vi "ExSubBin2x.vi"(2 "error in (no error)":errorcluster, 3 "Camera Handle":u32) -> (0 "error out":errorcluster, 1 "Camera Handle":u32)   [LabVIEW 2010]
panel:
  # "This is a SubVI that bins the CCD chip\nby 2 in both the x and y dimensions."
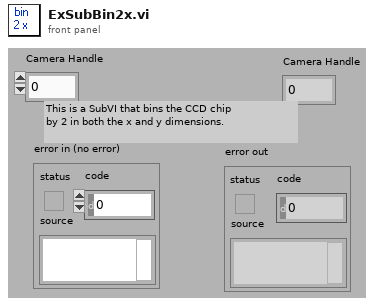
[diagram p1: front panel]
types:
  T1 = cluster{"X start":u32, "X end":u32, "X Binning/Grouping":u32, "Y start":u32, "Y end":u32, "Y Binning/Grouping":u32}
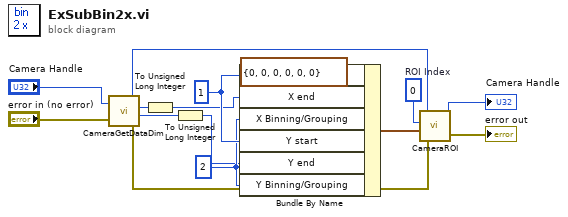
[diagram p0: block diagram]
diagram:
  w8 = u32 0  # ROI Index
  w6 = u32 2
  w7 = u32 1
  n1 = call <userlib>:"CameraGetDataDim.vi"("Camera Handle"="Camera Handle", "error in"="error in (no error)") -> ("Camera Handle"=w14:u32, "Xdim"=w5:u32, "Ydim"=w3:u32, "error out"=w12:errorcluster)
  n2 = To Unsigned Long Integer(number=w5) -> (unsigned 32bit integer=w4:u32)
  n3 = To Unsigned Long Integer(number=w3) -> (unsigned 32bit integer=w2:u32)
  n4 = Bundle By Name(cluster=T1 {"X start"=0, "X end"=0, "X Binning/Grouping"=0, "Y start"=0, "Y end"=0, "Y Binning/Grouping"=0} ("ROI Params"), "X start"=w7, "X end"=w4, "X Binning/Grouping"=w6, "Y start"=w7, "Y end"=w2, "Y Binning/Grouping"=w6) -> (w1:T1)
  n5 = call <userlib>:"CameraROI.vi"("error in"=w12, "ROI Params"=w1, "ROI Index"=w8, "Camera Handle"=w14) -> ("error out"=→"error out":errorcluster, "Camera Handle"=→"Camera Handle":u32)
